vi "Set Speed.vi"(8 "error in (no error)":errorcluster, 10 "speed":dbl, 11 "FLOM Settings in":T1={"VISA resource name"="", "Simulated?"=FALSE, "Pump Number"=1.0} {"Pump Number" min=1.0 max=20.0 step=1.0}) -> (0 "error out":errorcluster, 1 "Connection Error":bool, 3 "FLOM Settings out":T1={"VISA resource name"="", "Simulated?"=FALSE, "Pump Number"=1.0} {"Pump Number" min=1.0 max=20.0 step=1.0})   [LabVIEW 2018, in "FLOM Pump.lvlib"]
uses:
  FLOM Pump.lvlib
  Settings Cluster.ctl
panel:
  out "read buffer":string
  out "decimal integer string":string
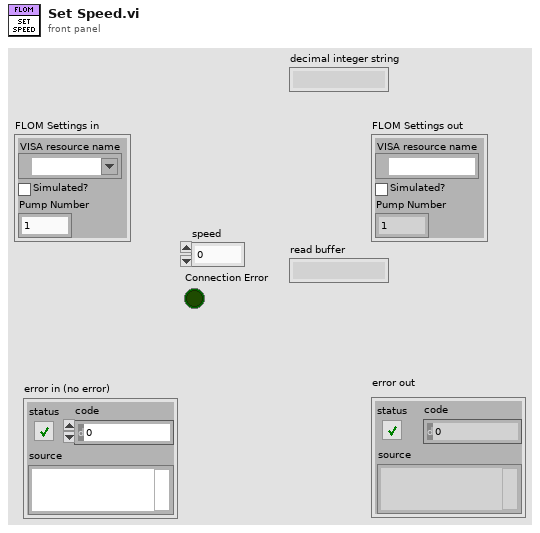
[diagram p1: front panel]
types:
  T1 = typedef "FLOM Pump.lvlib/Settings Cluster.ctl" = cluster{"VISA resource name":refnum<visa-resource-name>, "Simulated?":bool, "Pump Number":dbl}
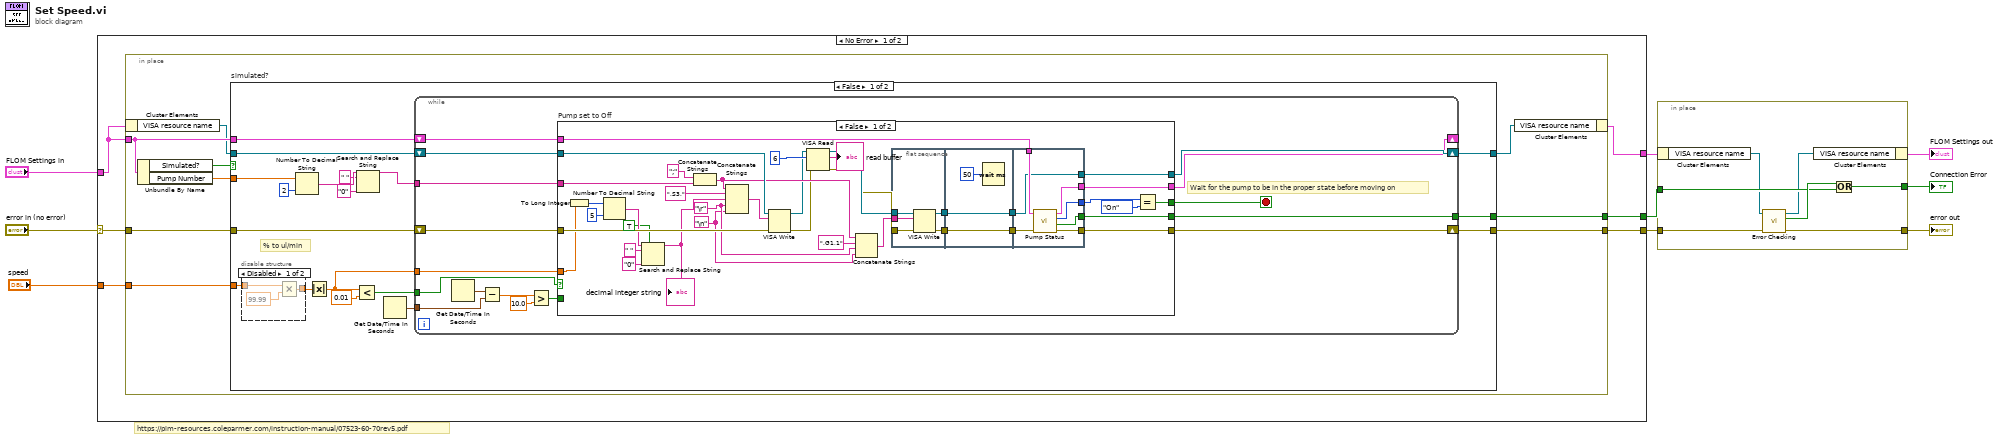
[diagram p0: block diagram]
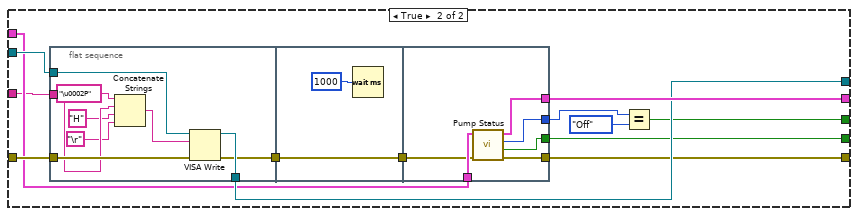
[diagram p3: hidden frame]
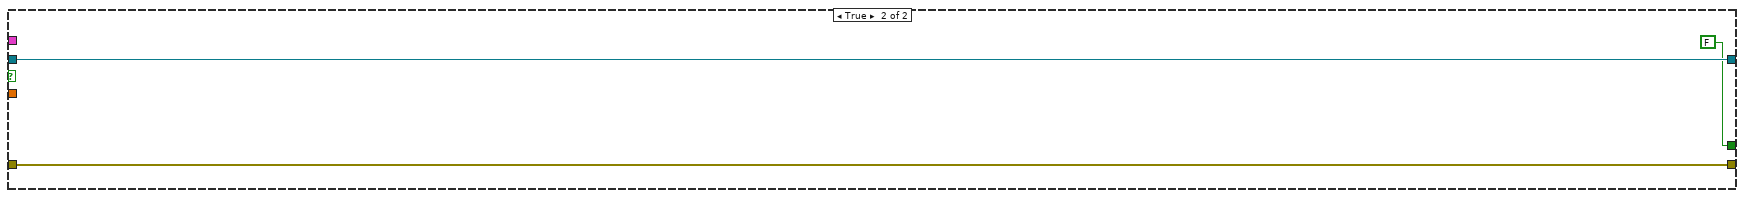
[diagram p4: hidden frame]
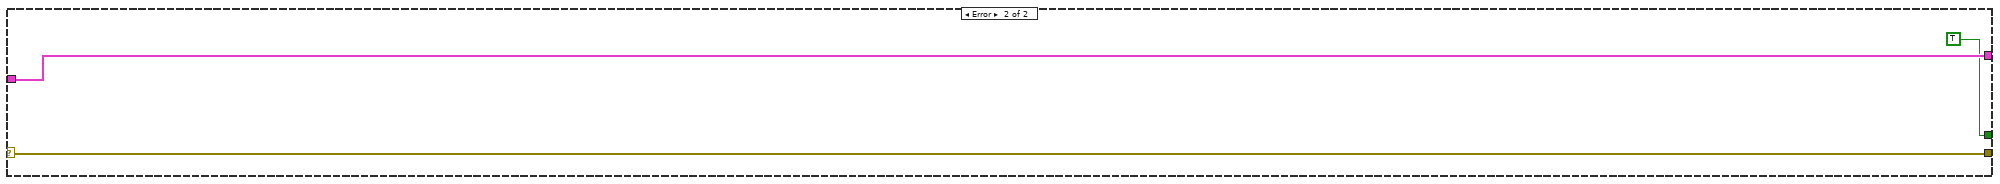
[diagram p5: hidden frame]
diagram:
  # "https://pim-resources.coleparmer.com/instruction-manual/07523-60-70rev5.pdf"
  n1 = case shown="No Error" "error in (no error)" {
    selector: "error in (no error)" -> [w15 w150]
    tunnel: [w14 w150] -> w9
    tunnel: [w10 w149] -> w2
    tunnel: "FLOM Settings in" -> [w11 w149]
    tunnel: "speed" -> [w13 _]
    tunnel: [w12 TRUE ("Connection Error")] -> w4
    frame No Error {
      n2 = in-place {
        in-place-border: w15 -> [w22]
        in-place-border: [w21] -> w14
        in-place-border: w13 -> [w20]
        in-place-border: w11 -> [w19]
        in-place-border: [w18] -> w12
        n3 = in-place-cluster #1(w11) -> ("VISA resource name"=w17:refnum<visa-resource-name>)
        n4 = Unbundle By Name(w19) -> ("Simulated?"=w24:bool, "Pump Number"=w23:dbl)
        n5 = case "simulated?" shown="False" w24 {
          tunnel: w22 -> [w35 w147]
          tunnel: [w40 w147] -> w21
          tunnel: w23 -> [w26 _]
          tunnel: w20 -> [w37 _]
          tunnel: w17 -> [w34 w146]
          tunnel: [w36 w146] -> w16
          tunnel: w19 -> [w32 _]
          tunnel: [w31 FALSE ("Connection Error")] -> w18
          frame False {
            # "% to ul/min"
            n6 = disable-structure shown="Disabled" {
              disable-tunnel: [w44 w46] -> w39
              disable-tunnel: w37 -> [w43 w46]
              frame Disabled {
                n7 = Multiply(x=w43, y=99.99) -> (x*y=w44:dbl)
              }
              frame Enabled {
              }
            }
            n8 = Number To Decimal String(number=w26, width (-)=i16 2) -> (decimal integer string=w29:string)
            n9 = Absolute Value(x=w39) -> (abs(x)=w38:dbl)
            n10 = Less?(x=w38, y=0.01) -> (x < y?=w41:bool)
            n11 = Search and Replace String(input string=w29, search string=" ", replace string="0" ("replace string (\"\")")) -> (result string=w25:string)  [unwired: 5 in, 3 out]
            n12 = Get Date/Time In Seconds() -> (seconds since 1Jan1904=w33:timestamp)
            n13 = while {
              tunnel: w41 -> [w62]
              tunnel: w38 -> [w60]
              tunnel: w25 -> [w51]
              shift-right: [w61] -> w40
              shift-left: w35 -> [w53]
              shift-right: [w59] -> w36
              shift-left: w34 -> [w52]
              tunnel: w33 -> [w55]
              shift-right: [w54] -> _
              shift-left: w32 -> [w50]
              tunnel: [w49] -> w31
              stop <- w47 stop-if-true
              # "Wait for the pump to be in the proper state before moving on"
              n14 = Get Date/Time In Seconds() -> (seconds since 1Jan1904=w58:timestamp)
              n15 = Subtract(x=w58, y=w55) -> (x-y=w56:dbl)
              n16 = Greater?(x=w56, y=10.0) -> (0:w48:bool)
              n17 = case "Pump set to Off" shown="False" w62 {
                tunnel: [w93 w121] -> w61
                tunnel: w60 -> [w65 _]
                tunnel: [w94 w123] -> w59
                tunnel: w51 -> [w81 w119]
                tunnel: w48 -> [_ _]
                tunnel: w50 -> [w92 w120]
                tunnel: [w91 w126] -> w54
                tunnel: w53 -> [w89 w127]
                tunnel: w52 -> [w90 w122]
                tunnel: [w88 w118] -> w49
                tunnel: [w85 w115] -> w47
                frame False {
                  w77 = "\n"
                  w78 = "\r"
                  n18 = To Long Integer(number=w65) -> (32bit integer=w64:i32)
                  n19 = Number To Decimal String(number=w64, width (-)=i16 5) -> (decimal integer string=w67:string)
                  n20 = Search and Replace String(replace all?=TRUE ("replace all? (F)"), input string=w67, search string=" ", replace string="0" ("replace string (\"\")")) -> (result string=w66:string)  [unwired: 4 in, 3 out]
                  "decimal integer string" <- w66
                  n21 = Concatenate Strings(";" ("string"), w81) -> (w80:string)
                  n22 = Concatenate Strings(w80, ",S3," ("string"), w66, w78, w77) -> (w99:string)
                  n23 = VISA Write(VISA resource name=w90, write buffer=w99, error in (no error)=w89) -> (VISA resource name out=w74:refnum<visa-resource-name>, error out=w72:errorcluster)  [unwired: 1 out]
                  n24 = VISA Read(VISA resource name=w74, byte count=u32 6, error in (no error)=w72) -> (VISA resource name out=w73:refnum<visa-resource-name>, read buffer=→"read buffer":string, error out=w71:errorcluster)  [unwired: 1 out]
                  n25 = Concatenate Strings(w80, ",G1,1" ("string"), w78, w77) -> (w84:string)
                  n26 = flat-sequence {
                    tunnel: w71 -> [w104]
                    tunnel: w84 -> [w103]
                    tunnel: w73 -> [w102]
                    tunnel: [w101] -> w98
                    tunnel: [w100] -> w95
                    tunnel: w98 -> [w106]
                    tunnel: [w106] -> w97
                    tunnel: [w105] -> w96
                    tunnel: w95 -> [w105]
                    tunnel: w97 -> [w111]
                    tunnel: w96 -> [w113]
                    tunnel: [w111] -> w94
                    tunnel: [w112] -> w93
                    tunnel: w92 -> [w114]
                    tunnel: [w108] -> w91
                    tunnel: [w110] -> w87
                    tunnel: [w109] -> w88
                    frame #0 {
                      n27 = VISA Write(VISA resource name=w102, write buffer=w103, error in (no error)=w104) -> (VISA resource name out=w101:refnum<visa-resource-name>, error out=w100:errorcluster)  [unwired: 1 out]
                    }
                    frame #1 {
                      n28 = Wait (ms)(milliseconds to wait=u32 50) -> ()  [unwired: 1 out]
                    }
                    frame #2 {
                      n29 = call "Pump Status.vi"("error in (no error)"=w113, "FLOM Settings In"=w114) -> ("error out"=w112:errorcluster, "Connection Error"=w109:bool, "Pump On?"=w110:enum16{"Off", "On", "Not Initialized"}, "FLOM Settings Out"=w108:T1)  [unwired: 4 in, 2 out]
                    }
                  }
                  n30 = Equal?(x=w87, y=enum16{"Off", "On", "Not Initialized"}."On") -> (x = y?=w85:bool)
                }
                frame True {
                  n31 = flat-sequence {
                    tunnel: w127 -> [w135]
                    tunnel: w122 -> [w134]
                    tunnel: w119 -> [w132]
                    tunnel: [w129] -> w123
                    tunnel: [w128] -> w124
                    tunnel: [w137] -> w125
                    tunnel: w124 -> [w137]
                    tunnel: w120 -> [w144]
                    tunnel: [w143] -> w117
                    tunnel: [w142] -> w126
                    tunnel: w125 -> [w141]
                    tunnel: [w140] -> w121
                    tunnel: [w139] -> w118
                    frame #0 {
                      n32 = Concatenate Strings("\u0002P" ("string"), w132, "H" ("string"), "\r") -> (w136:string)
                      n33 = VISA Write(VISA resource name=w134, write buffer=w136, error in (no error)=w135) -> (VISA resource name out=w129:refnum<visa-resource-name>, error out=w128:errorcluster)  [unwired: 1 out]
                    }
                    frame #1 {
                      n34 = Wait (ms)(milliseconds to wait=u32 1000) -> ()  [unwired: 1 out]
                    }
                    frame #2 {
                      n35 = call "Pump Status.vi"("error in (no error)"=w141, "FLOM Settings In"=w144) -> ("error out"=w140:errorcluster, "Connection Error"=w139:bool, "Pump On?"=w143:enum16{"Off", "On", "Not Initialized"}, "FLOM Settings Out"=w142:T1)  [unwired: 4 in, 2 out]
                    }
                  }
                  n36 = Equal?(x=w117, y=enum16{"Off", "On", "Not Initialized"}."Off") -> (x = y?=w115:bool)
                }
              }
            }
          }
          frame True {
          }
        }
        n37 = in-place-cluster #1("VISA resource name"=w16) -> (w10:T1)
      }
    }
    frame Error {
    }
  }
  n38 = in-place {
    in-place-border: w9 -> [w157]
    in-place-border: [w156] -> w8
    in-place-border: w4 -> [w154]
    in-place-border: [w153] -> w3
    n39 = in-place-cluster #2(w2) -> ("VISA resource name"=w152:refnum<visa-resource-name>)
    n40 = call "Error Checking.vi"("error in (no error)"=w157, "VISA resource name"=w152) -> ("error out"=w156:errorcluster, "Connection Error"=w155:bool, "VISA resource name"=w151:refnum<visa-resource-name>)  [unwired: 7 in]
    n41 = in-place-cluster #2("VISA resource name"=w151) -> (→"FLOM Settings out":T1)
    n42 = Or(x=w155, y=w154) -> (x .or. y?=w153:bool)
  }
  "error out" <- w8
  "Connection Error" <- w3
